vi "Compare.vi"(8 "error in":errorcluster, 10 "Actual":refnum<class "CANopen Response Message.lvclass">, 11 "SDO Response Compare Strategy in":refnum<class "SDO Response Compare Strategy.lvclass">) -> (0 "error out":errorcluster, 2 "Equal?":bool, 3 "SDO Response Compare Strategy out":refnum<class "SDO Response Compare Strategy.lvclass">)   [LabVIEW 2024, in "CANopen Master.lvlib" / "SDO Response Compare Strategy.lvclass"]
uses:
  SDO Response Compare Strategy.lvclass
  CANopen Response/CANopen Response Message.lvclass
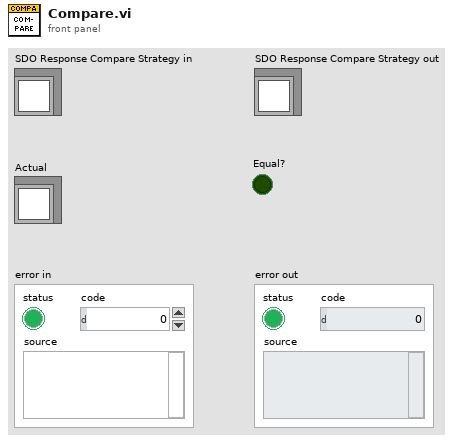
[diagram p1: front panel]
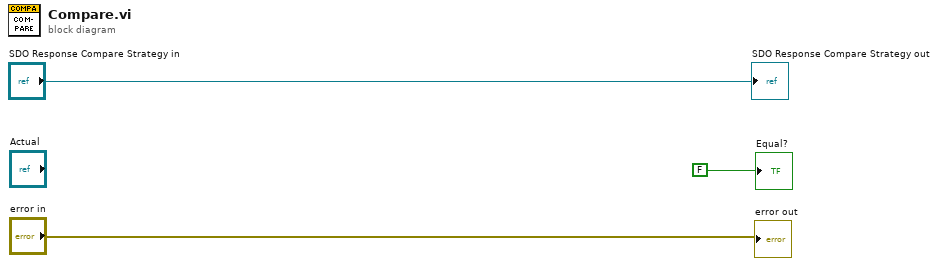
[diagram p0: block diagram]
diagram:
  "SDO Response Compare Strategy out" <- "SDO Response Compare Strategy in"
  "Equal?" <- FALSE ("Equal?")
  "error out" <- "error in"
